vi "Agilent 2000 3000 X-Series Jitter Analysis Histogram.vi"() -> ()   [LabVIEW 2015]
doc: "This example shows how to configure a histogram with a jitter measurement source and read histogram measurements.\n\n<b>Note:</b>\nThis example is specific to the 6000-X Series oscilloscopes. These features are not available on other models."
uses:
  Agilent 2000 3000 X-Series.lvlib
  Public/Configure/Jitter Analysis/Configure Jitter Measurement (N-Period to Period).vi
panel:
  in  "Delay For Histogram Data Acquisition (1000ms)":u32=1000
  out "Histogram Median":dbl
  out "Histogram Mean":dbl
  out "Histogram Mode":dbl
  out "Histogram Standard Deviation":dbl
  out "Histogram Hits in 1 Std Dev":dbl
  out "Histogram Hits in 2 Std Dev":dbl
  out "Histogram Hits in 3 Std Dev":dbl
  out "Histogram Total Hits":i32
  out "Histogram Peak-Peak Difference":dbl
  out "Histogram Min Bin Hit":dbl
  out "Histogram Max Bin Hit":dbl
  out "Histogram Bin Width":dbl
  out "Histogram Peak Hits":i32
  in  "Histogram Type (0: Vertical)":i32(ring) items=["Vertical", "Horizontal", "Measurement"]
  in  "Histogram Source (0: Channel 1)":u16(ring)=13 items=["Channel 1", "Channel 2", "Channel 3", "Channel 4", "Math 1", "Math 2", "Math 3", "Math 4", "Reference Waveform 1", "Reference Waveform 2", "Reference Waveform 3", "Reference Waveform 4", "Color Grade", "Measurement 1", "Measurement 2", "Measurement 3", "Measurement 4", "Measurement 5", "Measurement 6", "Measurement 7", "Measurement 8", "Measurement 9", "Measurement 10"]
  in  "Enable Jitter Trend (F: Disable)":bool
  in  "Jitter Source (1: Measurement1)":i32(ring)=1 items=["Measurement 1"=1, "Measurement 2"=2, "Measurement 3"=3, "Measurement 4"=4, "Measurement 5"=5, "Measurement 6"=6, "Measurement 7"=7, "Measurement 8"=8, "Measurement 9"=9, "Measurement 10"=10]
  in  "Enable Jitter Histogram (F: Disable)":bool=TRUE
  in  "Enable Jitter Spectrum (F: Disable)":bool
  in  "N-Period to Period Slope (0: Rising)":u16(ring) items=["Rising", "Falling"]
  in  "N-Period to Period Source (0: Channel 1)":u16(ring) items=["Channel 1", "Channel 2", "Channel 3", "Channel 4", "Math 1", "Math 2", "Math 3", "Math 4", "Reference Waveform 1", "Reference Waveform 2", "Reference Waveform 3", "Reference Waveform 4"]
  in  "Number of Periods (1)":i32=2
  in  "Enable Output (F: Disable)":bool=TRUE
  in  "Waveform Generator Number (1: Waveform Generator 1)":i32(ring)=2 items=["Waveform Generator 1"=1, "Waveform Generator 2"=2]
  in  "Frequency (1000 Hz)":dbl=10000000.0
  in  "Function Type (0: Sine)":i32(ring)=1 items=["Sine", "Square", "Ramp", "Pulse", "Noise", "DC", "Sine Cardinal", "Exponential Rise", "Exponential Fall", "Cardiac", "Gaussian Pulse", "Arbitrary"]
  in  "VISA resource name":refnum<visa-resource-name>
  # "(c) 2011-2023 National Instruments.  ALL RIGHTS RESERVED."
  # "N-Period to Period Measurement Configuration"
  # "Wave Generator Configuration"
  # "Histogram Measurements"
  # "Jitter Analysis Configuration"
  # "Histogram Configuration"
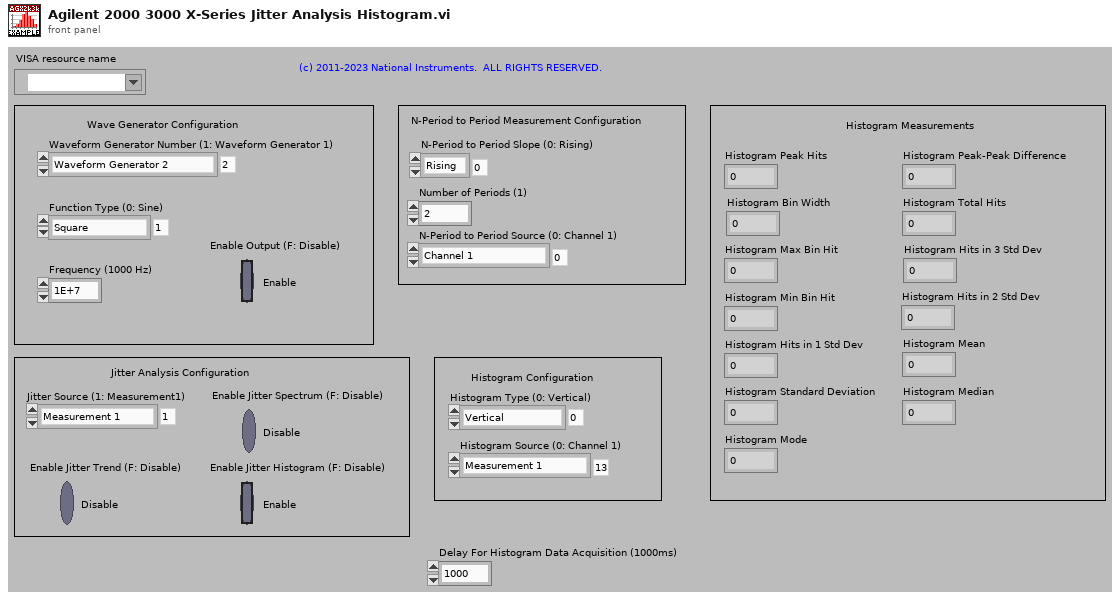
[diagram p1: front panel]
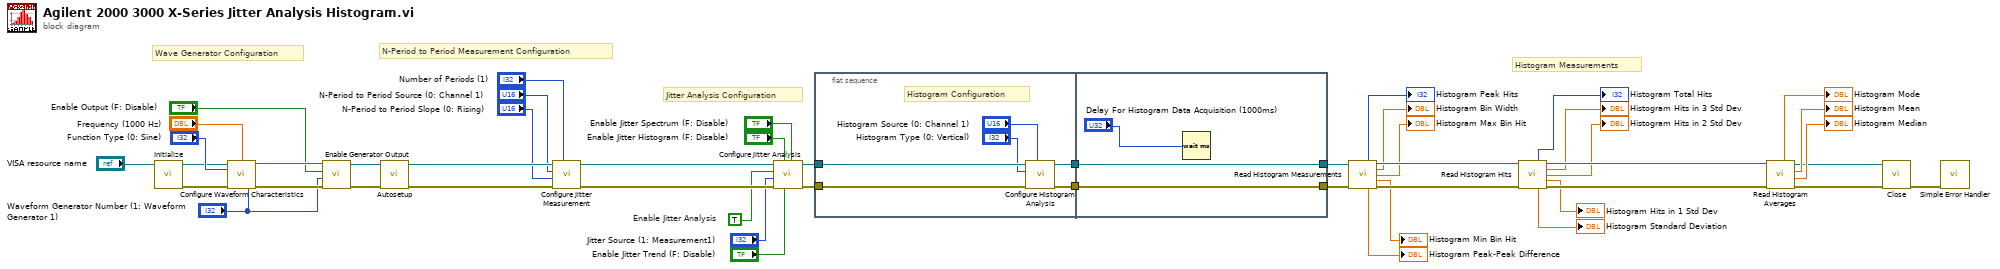
[diagram p0: block diagram]
diagram:
  w26 = TRUE  # Enable Jitter Analysis
  # "Histogram Measurements"
  # "Jitter Analysis Configuration"
  # "N-Period to Period Measurement Configuration"
  # "Wave Generator Configuration"
  n1 = call "Initialize.vi"("VISA resource name"="VISA resource name") -> ("error out"=w41:errorcluster, "VISA resource name out"=w40:refnum<visa-resource-name>)  [unwired: 9 in]
  n2 = call "Configure Waveform Characteristics.vi"("VISA resource name"=w40, "Frequency (1000 Hz)"="Frequency (1000 Hz)", "Function Type (0: Sine)"="Function Type (0: Sine)", "error in (no error)"=w41, "Waveform Generator Number (1: Waveform Generator 1)"="Waveform Generator Number (1: Waveform Generator 1)") -> ("VISA resource name out"=w48:refnum<visa-resource-name>, "error out"=w47:errorcluster)  [unwired: 9 in]
  n3 = call "Enable Generator Output.vi"("error in (no error)"=w47, "Waveform Generator Number (1: Waveform Generator 1)"="Waveform Generator Number (1: Waveform Generator 1)", "Enable Output (F: Disable)"="Enable Output (F: Disable)", "VISA resource name"=w48) -> ("error out"=w45:errorcluster, "VISA resource name out"=w46:refnum<visa-resource-name>)  [unwired: 6 in]
  n4 = call "Autosetup.vi"("error in (no error)"=w45, "VISA resource name"=w46) -> ("error out"=w36:errorcluster, "VISA resource name out"=w37:refnum<visa-resource-name>)  [unwired: 8 in]
  n5 = call-poly "Configure Jitter Measurement.vi"("Number of Periods (1)"="Number of Periods (1)", "error in (no error)"=w36, "N-Period to Period Slope (0: Rising)"="N-Period to Period Slope (0: Rising)", "N-Period to Period Source (0: Channel 1)"="N-Period to Period Source (0: Channel 1)", "VISA resource name"=w37) -> ("error out"=w31:errorcluster, "VISA resource name out"=w32:refnum<visa-resource-name>)  [unwired: 5 in]
  n6 = call "Configure Jitter Analysis.vi"("Enable Jitter Spectrum (F: Disable)"="Enable Jitter Spectrum (F: Disable)", "Enable Jitter Trend (F: Disable)"="Enable Jitter Trend (F: Disable)", "Enable Jitter Histogram (F: Disable)"="Enable Jitter Histogram (F: Disable)", "error in (no error)"=w31, "Jitter Source (1: Measurement1)"="Jitter Source (1: Measurement1)", "Enable Jitter Analysis (T: Enable)"=w26, "VISA resource name"=w32) -> ("error out"=w24:errorcluster, "VISA resource name out"=w25:refnum<visa-resource-name>)  [unwired: 3 in]
  n7 = flat-sequence {
    tunnel: w25 -> [w55]
    tunnel: w24 -> [w54]
    tunnel: [w51] -> w4
    tunnel: [w50] -> w3
    tunnel: [w57] -> w22
    tunnel: [w58] -> w23
    tunnel: w4 -> [w58]
    tunnel: w3 -> [w57]
    frame #0 {
      # "Histogram Configuration"
      n8 = call "Configure Histogram Analysis.vi"("Histogram Source (0: Channel 1)"="Histogram Source (0: Channel 1)", "error in (no error)"=w54, "Histogram Type (0: Vertical)"="Histogram Type (0: Vertical)", "VISA resource name"=w55) -> ("error out"=w50:errorcluster, "VISA resource name out"=w51:refnum<visa-resource-name>)  [unwired: 6 in]
    }
    frame #1 {
      n9 = Wait (ms)(milliseconds to wait="Delay For Histogram Data Acquisition (1000ms)") -> ()  [unwired: 1 out]
    }
  }
  n10 = call "Read Histogram Measurements.vi"("VISA resource name"=w23, "error in (no error)"=w22) -> ("Histogram Peak Hits"=→"Histogram Peak Hits":i32, "VISA resource name out"=w21:refnum<visa-resource-name>, "Histogram Bin Width"=→"Histogram Bin Width":dbl, "Histogram Max Bin Hit"=→"Histogram Max Bin Hit":dbl, "Histogram Min Bin Hit"=→"Histogram Min Bin Hit":dbl, "Histogram Peak-Peak Difference"=→"Histogram Peak-Peak Difference":dbl, "error out"=w20:errorcluster)  [unwired: 7 in]
  n11 = call "Read Histogram Hits.vi"("VISA resource name"=w21, "error in (no error)"=w20) -> ("Histogram Total Hits"=→"Histogram Total Hits":i32, "VISA resource name out"=w19:refnum<visa-resource-name>, "Histogram Hits in 3 Std Dev"=→"Histogram Hits in 3 Std Dev":dbl, "Histogram Hits in 2 Std Dev"=→"Histogram Hits in 2 Std Dev":dbl, "Histogram Hits in 1 Std Dev"=→"Histogram Hits in 1 Std Dev":dbl, "Histogram Standard Deviation"=→"Histogram Standard Deviation":dbl, "error out"=w18:errorcluster)  [unwired: 7 in]
  n12 = call "Read Histogram Averages.vi"("error in (no error)"=w18, "VISA resource name"=w19) -> ("error out"=w1:errorcluster, "Histogram Median"=→"Histogram Median":dbl, "Histogram Mean"=→"Histogram Mean":dbl, "VISA resource name out"=w2:refnum<visa-resource-name>, "Histogram Mode"=→"Histogram Mode":dbl)  [unwired: 5 in]
  n13 = call "Close.vi"("error in (no error)"=w1, "VISA resource name"=w2) -> ("error out"=w49:errorcluster)  [unwired: 9 in]
  n14 = call <vilib>:"Simple Error Handler.vi"("error in (no error)"=w49) -> ()  [unwired: 4 in, 5 out]
